vi "Get Command.vi"(8 "error in (no error)":errorcluster, 11 "RFFE RegReadExtLong Command in":refnum<class "RFFE RegReadExtLong Command.lvclass">) -> (0 "error out":errorcluster, 2 "Command":u8=12 format="%02x", 3 "RFFE RegReadExtLong Command out":refnum<class "RFFE RegReadExtLong Command.lvclass">)   [LabVIEW 2018, in "MIPI RFFE API.lvlib" / "RFFE RegReadExtLong Command.lvclass"]
uses:
  RFFE RegReadExtLong Command.lvclass
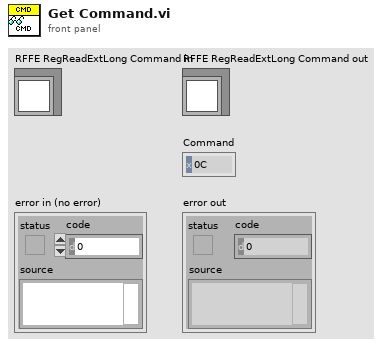
[diagram p1: front panel]
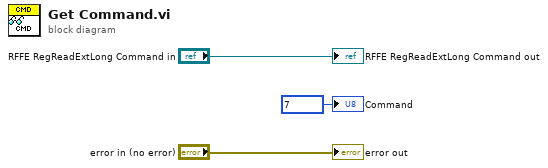
[diagram p0: block diagram]
diagram:
  "error out" <- "error in (no error)"
  "RFFE RegReadExtLong Command out" <- "RFFE RegReadExtLong Command in"
  "Command" <- u8 7 ("Command")
